vi "Start Trigger TIO.vi"(8 "error in":errorcluster) -> (0 "error out":errorcluster, 3 "Trigger task ID out":u32 format="%.0x")   [LabVIEW 2009]
uses:
  Acquisition Settings.vi
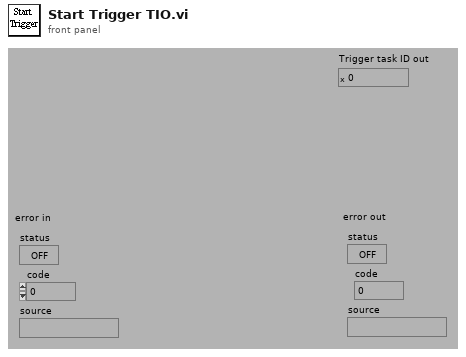
[diagram p1: front panel]
types:
  T1 = cluster{"Device Number":i16, "Counter Number":i16, "Signal Routing Configuration":i16}
  T2 = cluster{"Name":string, "Signal Routing":cluster{"signal name":u16, "signal source":u16, "signal source line number":u32, "signal name line number":u32}[]}[]
  T3 = cluster{"Name":string, "Signal Routing":cluster{"signal name":u16, "signal source":u16, "signal source line number":u32, "signal name line number":u32}[]}
  T4 = cluster{"signal name":u16, "signal source":u16, "signal source line number":u32, "signal name line number":u32}[]
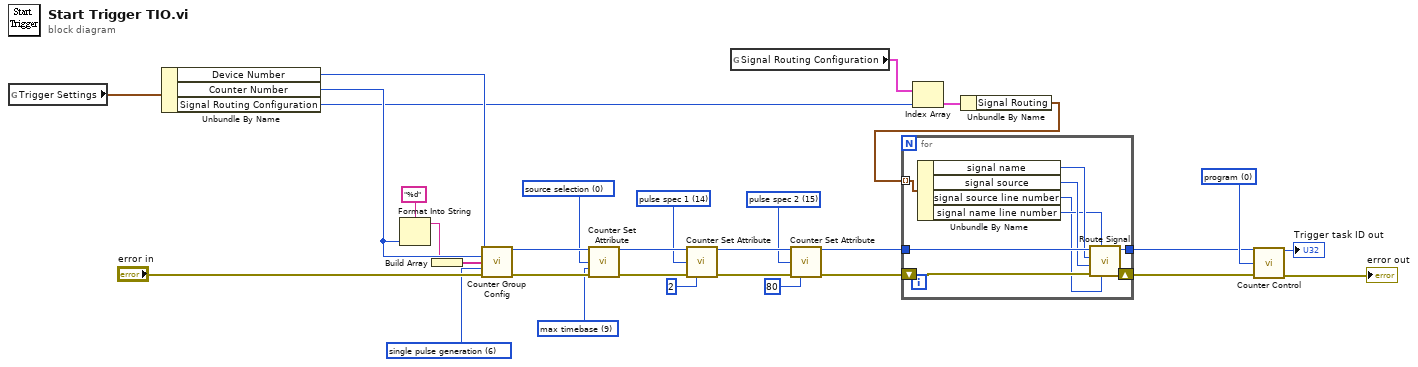
[diagram p0: block diagram]
diagram:
  w10 = u32 6 items=["simple event counting", "single period measurement", "single pulse width measurement", "triggered pulse width measurement", "two signal edge separation measurement", "position measurement", "single pulse generation", "single triggered pulse generation", "retriggerable pulse generation", "pulse train generation", "frequency shift keying", "buffered event counting", "buffered period measurement", "buffered semiperiod measurement", "buffered pulse width measurement", "buffered two signal edge separation measurement", "buffered position measurement"] ("task type")
  w15 = u32 15 items=["source selection", "source polarity", "gate selection", "gate polarity", "output mode", "output polarity", "aux line selection", "aux line polarity", "start trigger", "counting synchronous", "up down", "buffer mode", "encoder type", "initial count", "pulse spec 1", "pulse spec 2", "pulse spec 3", "pulse spec 4", "auto increment", "prescale value", "Z index active", "Z index value"] ("attribute ID")
  w17 = u32 14 items=["source selection", "source polarity", "gate selection", "gate polarity", "output mode", "output polarity", "aux line selection", "aux line polarity", "start trigger", "counting synchronous", "up down", "buffer mode", "encoder type", "initial count", "pulse spec 1", "pulse spec 2", "pulse spec 3", "pulse spec 4", "auto increment", "prescale value", "Z index active", "Z index value"] ("attribute ID")
  w18 = u32 9 items=["yes", "no", "positive", "negative", "high", "low", "low to high", "high to low", "default", "max timebase", "other counter gate", "other counter TC", "other counter output", "other counter source", "source", "gate", "aux line", "in start trigger", "in stop trigger", "automatic", "enabled", "count up", "count down", "hardware", "single", "double", "pulse", "toggle", "quadrature encoder X1", "quadrature encoder X2", "quadrature encoder X4", "two pulse counting", "A high B high", "A high B low", "A low B high", "A low B low", "PFI n", "RTSI n", "timebase n"] ("attribute value type")
  w19 = u32 0 items=["source selection", "source polarity", "gate selection", "gate polarity", "output mode", "output polarity", "aux line selection", "aux line polarity", "start trigger", "counting synchronous", "up down", "buffer mode", "encoder type", "initial count", "pulse spec 1", "pulse spec 2", "pulse spec 3", "pulse spec 4", "auto increment", "prescale value", "Z index active", "Z index value"] ("attribute ID")
  w29 = u32 0 items=["program", "reset", "arm", "prepare", "disarm", "count up", "count down", "switch cycle", "snapshot"] ("control code")
  n1 = global read "Acquisition Settings.vi" "Trigger Settings"() -> (w9:T1)
  n2 = Unbundle By Name(w9) -> ("Device Number"=w28:i16, "Counter Number"=w26:i16, "Signal Routing Configuration"=w2:i16)
  n3 = Format Into String(format string="%d" ("Format String"), w26) -> (resulting string=w12:string)  [unwired: 2 in, 1 out]
  n4 = Build Array(w12) -> (w13:string[])
  n5 = call <vilib>:"Counter Group Config.vi"("device"=w28, "group"=w26, "counter list"=w13, "task type"=w10, "error in (no error)"="error in") -> ("task ID"=w25:u32, "error out"=w24:errorcluster)  [unwired: 8 in, 1 out]
  n6 = call <vilib>:"Counter Set Attribute.vi"("task ID in"=w25, "attribute ID"=w19, "attribute value type"=w18, "error in (no error)"=w24) -> ("task ID out"=w22:u32, "error out"=w23:errorcluster)  [unwired: 10 in]
  n7 = call <vilib>:"Counter Set Attribute.vi"("task ID in"=w22, "attribute ID"=w17, "error in (no error)"=w23, "attribute value number"=u32 2) -> ("task ID out"=w21:u32, "error out"=w20:errorcluster)  [unwired: 10 in]
  n8 = global read "Acquisition Settings.vi" "Signal Routing Configuration"() -> (w1:T2)
  n9 = call <vilib>:"Counter Set Attribute.vi"("task ID in"=w21, "attribute ID"=w15, "error in (no error)"=w20, "attribute value number"=u32 80) -> ("task ID out"=w6:u32, "error out"=w5:errorcluster)  [unwired: 10 in]
  n10 = Index Array(array=w1, index=w2) -> (element=w8:T3)
  n11 = Unbundle By Name(w8) -> ("Signal Routing"=w7:T4)
  n12 = for {
    tunnel: w6 -> [w40]
    shift-right: [w32] -> w3
    shift-left: w5 -> [w39]
    tunnel: w7 -> [w38] mode=indexing
    tunnel: [w33] -> w4
    n13 = Unbundle By Name(w38) -> ("signal name"=w37:u16, "signal source"=w36:u16, "signal source line number"=w34:u32, "signal name line number"=w35:u32)
    n14 = call <vilib>:"Route Signal.vi"("signal source line number"=w34, "signal name line number"=w35, "error in (no error)"=w39, "signal source"=w36, "signal name"=w37, "task ID"=w40) -> ("error out"=w32:errorcluster, "task ID out"=w33:u32)  [unwired: 4 in]
  }
  n15 = call <vilib>:"Counter Control.vi"("task ID"=w4, "control code"=w29, "error in (no error)"=w3) -> ("task ID out"=→"Trigger task ID out":u32, "error out"=→"error out":errorcluster)  [unwired: 11 in]
